vi "resetGraphs.vi"(8 "error in (no error)":errorcluster, 11 "AnalysisResultsViewer in":refnum<class "AnalysisResultsViewer.lvclass">) -> (0 "error out":errorcluster, 3 "AnalysisResultsViewer out":refnum<class "AnalysisResultsViewer.lvclass">)   [LabVIEW 2011, in "Views.lvlib" / "Camera.lvlib" / "AnalysisResultsViewer.lvclass"]
uses:
  AnalysisResultsViewer.lvclass
  AnalysisResultsViewer.lvclass/AnalysisResultsViewer.ctl
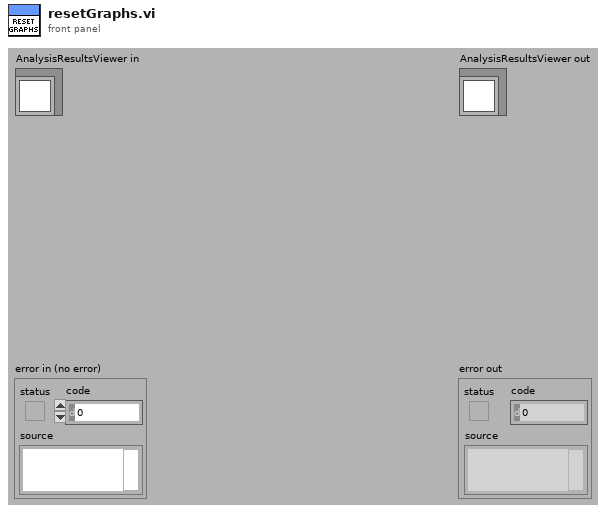
[diagram p1: front panel]
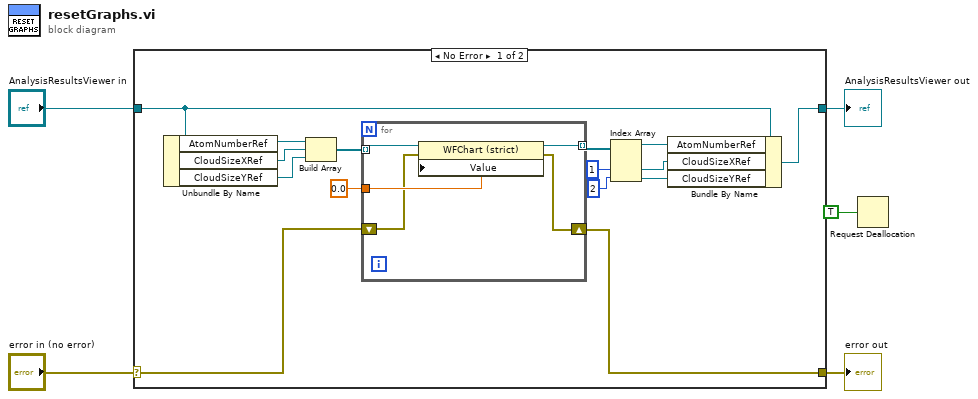
[diagram p0: block diagram]
diagram:
  n1 = case shown="No Error" "error in (no error)" {
    selector: "error in (no error)" -> [w15 w27]
    tunnel: [w14 w27] -> w4
    tunnel: [w12 w26] -> w2
    tunnel: "AnalysisResultsViewer in" -> [w13 w26]
    frame No Error {
      n2 = Unbundle By Name(w13) -> ("AtomNumberRef"=w20:refnum<vi>, "CloudSizeXRef"=w19:refnum<vi>, "CloudSizeYRef"=w18:refnum<vi>)
      n3 = Build Array(w20, w19, w18) -> (w17:refnum<vi>[])
      n4 = for {
        tunnel: w17 -> [w25] mode=indexing
        tunnel: 0.0 -> [w24]
        tunnel: [w21] -> w11 mode=indexing
        shift-right: [w22] -> w14
        shift-left: w15 -> [w23]
        n5 = property class="WFChart (strict)"(reference=w25, error in=w23, "Value"=w24) -> (reference out=w21:refnum<vi>, error out=w22:errorcluster)
      }
      n6 = Index Array(array=w11, index #2=1, index #3=2) -> (element #1=w10:refnum<vi>, element #2=w8:refnum<vi>, element #3=w9:refnum<vi>)  [unwired: 1 in]
      n7 = Bundle By Name(cluster=w13, "AtomNumberRef"=w10, "CloudSizeXRef"=w8, "CloudSizeYRef"=w9) -> (w12:refnum<class "AnalysisResultsViewer.lvclass">)
    }
    frame Error {
    }
  }
  "error out" <- w4
  "AnalysisResultsViewer out" <- w2
  n8 = Request Deallocation(TRUE ("flag")) -> ()
